vi "uTransport_Queue_SendMsg.vi"(8 "error in (no error)":errorcluster, 10 "Msg":refnum<class "uMsg.lvclass">, 11 "uTransport_Queue in":refnum<class "uTransport_Queue.lvclass">) -> (0 "error out":errorcluster, 3 "uTransport_Queue out":refnum<class "uTransport_Queue.lvclass">)   [LabVIEW 2021, in "uFramework.lvlib" / "uTransport_Queue.lvclass"]
uses:
  uTransport_Queue.lvclass
  uMsg/uMsg.lvclass
  uTransport_Queue.lvclass/uTransport_Queue.ctl
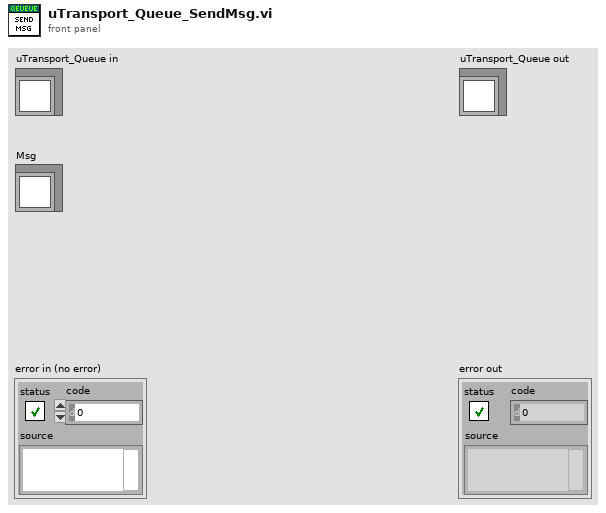
[diagram p1: front panel]
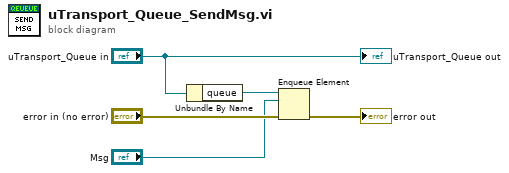
[diagram p0: block diagram]
diagram:
  n1 = Unbundle By Name("uTransport_Queue in") -> ("queue"=w4:refnum<queue>)
  n2 = Enqueue Element(queue=w4, element="Msg", error in (no error)="error in (no error)") -> (error out=→"error out":errorcluster)  [unwired: 1 in, 2 out]
  "uTransport_Queue out" <- "uTransport_Queue in"
